vi "Command-DeleteDVR.vi"(8 "error in (no error)":errorcluster, 10 "Data":T1, 11 "Engine in":refnum<class "Engine.lvclass">) -> (0 "error out":errorcluster, 3 "Engine out":refnum<class "Engine.lvclass">)   [LabVIEW 2024, in "GLF.lvlib" / "Engine.lvclass"]
uses:
  Engine.lvclass
  Engine.lvclass/Engine.ctl
  Window/Window.lvclass
  IAmGLF/IAmGLF.lvclass
  Command-DeleteDVR--cluster.ctl
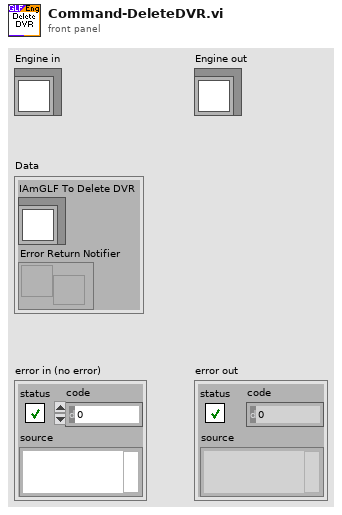
[diagram p1: front panel]
types:
  T1 = typedef "GLF.lvlib/Engine.lvclass/Command-DeleteDVR--cluster.ctl" = cluster{"IAmGLF To Delete DVR":refnum<class "IAmGLF.lvclass">, "Error Return Notifier":refnum<notifier>}
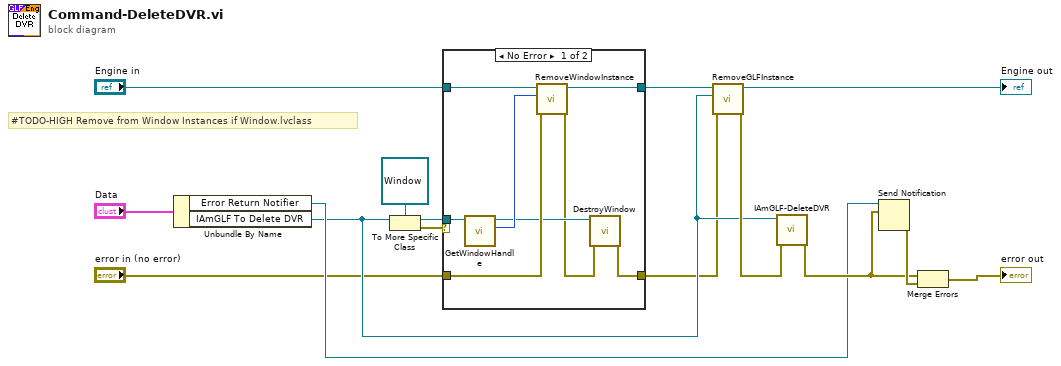
[diagram p0: block diagram]
diagram:
  # "#TODO-HIGH Remove from Window Instances if Window.lvclass"
  n1 = Unbundle By Name("Data") -> ("Error Return Notifier"=w8:refnum<notifier>, "IAmGLF To Delete DVR"=w7:refnum<class "IAmGLF.lvclass">)
  n2 = To More Specific Class(target class=refnum<class "Window.lvclass"> refnum ("GLF.lvlib:Window.lvclass"), reference=w7) -> (specific class reference=w6:refnum<class "Window.lvclass">, error out=w1:errorcluster)  [unwired: 1 in]
  n3 = case shown="No Error" w1 {
    tunnel: w6 -> [w23 _]
    tunnel: "Engine in" -> [w22 w25]
    tunnel: "error in (no error)" -> [w20 w24]
    tunnel: [w19 w25] -> w3
    tunnel: [w16 w24] -> w2
    frame No Error {
      n4 = call "GetWindowHandle.vi"("Window in"=w23) -> ("SDL_Window *"=w21:i64, "Window out"=w18:refnum<class "Window.lvclass">)  [unwired: 9 in]
      n5 = call "RemoveWindowInstance.vi"("error in (no error)"=w20, "SDL_Window *"=w21, "Engine in"=w22) -> ("error out"=w17:errorcluster, "Engine out"=w19:refnum<class "Engine.lvclass">)  [unwired: 6 in, 1 out]
      n6 = call "DestroyWindow.vi"("error in (no error)"=w17, "Window in"=w18) -> ("error out"=w16:errorcluster)  [unwired: 8 in, 1 out]
    }
    frame Error {
    }
  }
  n7 = call "RemoveGLFInstance.vi"("error in (no error)"=w2, "GLF Instance"=w7, "Engine in"=w3) -> ("error out"=w15:errorcluster, "Engine out"=→"Engine out":refnum<class "Engine.lvclass">)  [unwired: 7 in]
  n8 = call-dynamic "IAmGLF-DeleteDVR.vi"("error in (no error)"=w15, "IAmGLF in"=w7) -> ("error out"=w13:errorcluster)  [unwired: 8 in, 1 out]
  n9 = Send Notification(notification=w13, notifier=w8) -> (error out=w14:errorcluster)  [unwired: 1 in, 1 out]
  n10 = Merge Errors(w13, w14) -> (→"error out":errorcluster)
